vi "SUB.vi"() -> ()   [LabVIEW 2018]
uses:
  Channel Sub/Channel Sub.lvclass
  C:/Users/Denis/Desktop/communication-manager/communication-manager/Communication Channel/Communication Channel.lvclass
  RxTx/RxTx.lvclass
  <vilib>/addons/zeromq/zmq_context.lvclass
  Communication Channel/Communication Channel.lvclass
panel:
  out "error out":errorcluster
  out "Received message":string
  in  "RxTx in 2":refnum<class "RxTx.lvclass">
  in  "Stop App":bool
  in  "Channel Sub.lvclass":refnum<class "Channel Sub.lvclass">
  # "SUBSCRIBE example"
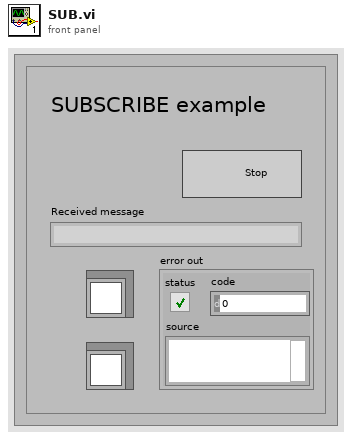
[diagram p1: front panel]
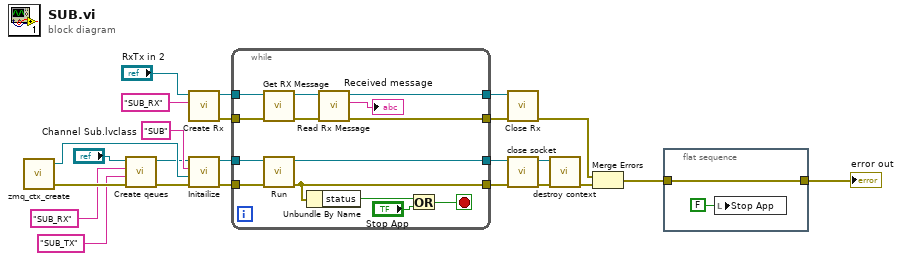
[diagram p0: block diagram]
diagram:
  n1 = call <vilib>:"zmq_ctx_create.vi"() -> ("error out"=w23:errorcluster, "context out"=w24:refnum<class "zmq_context.lvclass">)  [unwired: 4 in]
  n2 = call "Create qeues.vi"("error in (no error)"=w23, "name qeue Tx"="SUB_TX" ("name qeue Rx"), "name qeue Rx"="SUB_RX", "Communication Channel in"="Channel Sub.lvclass") -> ("error out"=w19:errorcluster, "Communication Channel out"=w20:refnum<class "Channel Sub.lvclass">)  [unwired: 6 in]
  n3 = call "Create Rx.vi"("Reader Name"="SUB_RX" ("Writer Name"), "RxTx in"="RxTx in 2") -> ("error out"=w11:errorcluster, "RxTx out"=w12:refnum<class "RxTx.lvclass">)  [unwired: 8 in]
  n4 = call-dynamic "Initailize.vi"("error in (no error)"=w19, "zeromq.lvlib:ZeroMQ Context"=w24, "Name"="SUB", "Channel Sub in"=w20) -> ("error out"=w15:errorcluster, "Channel Sub out"=w16:refnum<class "Channel Sub.lvclass">)  [unwired: 6 in]
  n5 = while {
    tunnel: w16 -> [w31]
    tunnel: w15 -> [w30]
    tunnel: [w29] -> w14
    tunnel: [w28] -> w13
    tunnel: w12 -> [w38]
    tunnel: w11 -> [w37]
    tunnel: [w34] -> w10
    tunnel: [w33] -> w9
    stop <- w25 stop-if-true
    n6 = call "Get RX Message.vi"("error in (no error)"=w37, "RxTx in"=w38) -> ("error out"=w35:errorcluster, "RxTx out"=w36:refnum<class "RxTx.lvclass">)  [unwired: 7 in, 1 out]
    n7 = call-dynamic "Run.vi"("error in (no error)"=w30, "Channel Sub in"=w31) -> ("error out"=w28:errorcluster, "Channel Sub out"=w29:refnum<class "Channel Sub.lvclass">)  [unwired: 8 in]
    n8 = Unbundle By Name(w28) -> ("status"=w27:bool)
    n9 = call "Read Rx Message.vi"("error in (no error)"=w35, "RxTx in"=w36) -> ("error out"=w34:errorcluster, "Rx Message"=→"Received message":string, "RxTx out"=w33:refnum<class "RxTx.lvclass">)  [unwired: 7 in]
    n10 = Or(x=w27, y="Stop App") -> (x .or. y?=w25:bool)
  }
  n11 = call "Close Rx.vi"("error in (no error)"=w10, "RxTx in"=w9) -> ("error out"=w3:errorcluster)  [unwired: 8 in, 1 out]
  n12 = call "close socket.vi"("error in (no error)"=w13, "Communication Channel in"=w14) -> ("error out"=w5:errorcluster, "Communication Channel out"=w6:refnum<class "Channel Sub.lvclass">)  [unwired: 8 in]
  n13 = call "destroy context.vi"("error in (no error)"=w5, "Communication Channel in"=w6) -> ("error out"=w4:errorcluster)  [unwired: 8 in, 1 out]
  n14 = Merge Errors(w3, w4) -> (w2:errorcluster)
  n15 = flat-sequence {
    tunnel: w2 -> [w40]
    tunnel: [w40] -> w1
    frame #0 {
      n16 = local write "Stop App"(FALSE ("Stop App")) -> ()
    }
  }
  "error out" <- w1
